vi "SVA 4MV6 P001 CCE.vi"() -> ()   [LabVIEW 2020]
doc: "Ceballos Conde Emanuel 4MV6 Sistemas de visión artificial 2022/1\nEste vi permite obtener el gradiente en x , gradiente en Y o gradiente general en susecion de una serie de imagenes ubicadas en una carpeta , si se utiliza como subvi la salida obtenida sera el gradiente da la ultima imagen de la carpeta."
uses:
  <vilib>/userDefined/High Color/IMAQdx.ctl
  <vilib>/vision/driver/IMAQdx.llb/IMAQdx Buffer Number Mode.ctl
  <vilib>/vision/driver/NI_Vision_Acquisition_Software.lvlib
panel:
  out "Cal Dis":bool
  out "CII":bool
  out "CID":bool
  in  "recalcular distancia":bool
  in  "recapturar imagen izquierda":bool
  in  "recapturar Imagen derecha":bool
  in  "capturar":bool
  out "Imagen izquierda":T1(plugin-control)
  out "video":T1(plugin-control)
  in  "stop":bool
  in  "Session In":T2
  out "Bcx":u32
  out "Bcy":u32
  out "Gcx":u32
  out "Gcy":u32
  out "Rcy":u32
  out "Rcx":u32
  out "Imagen derecha":T1(plugin-control)
  # "Ceballos Conde Emanuel\n4MV6\nSistemas de visión artificial\n2022/1"
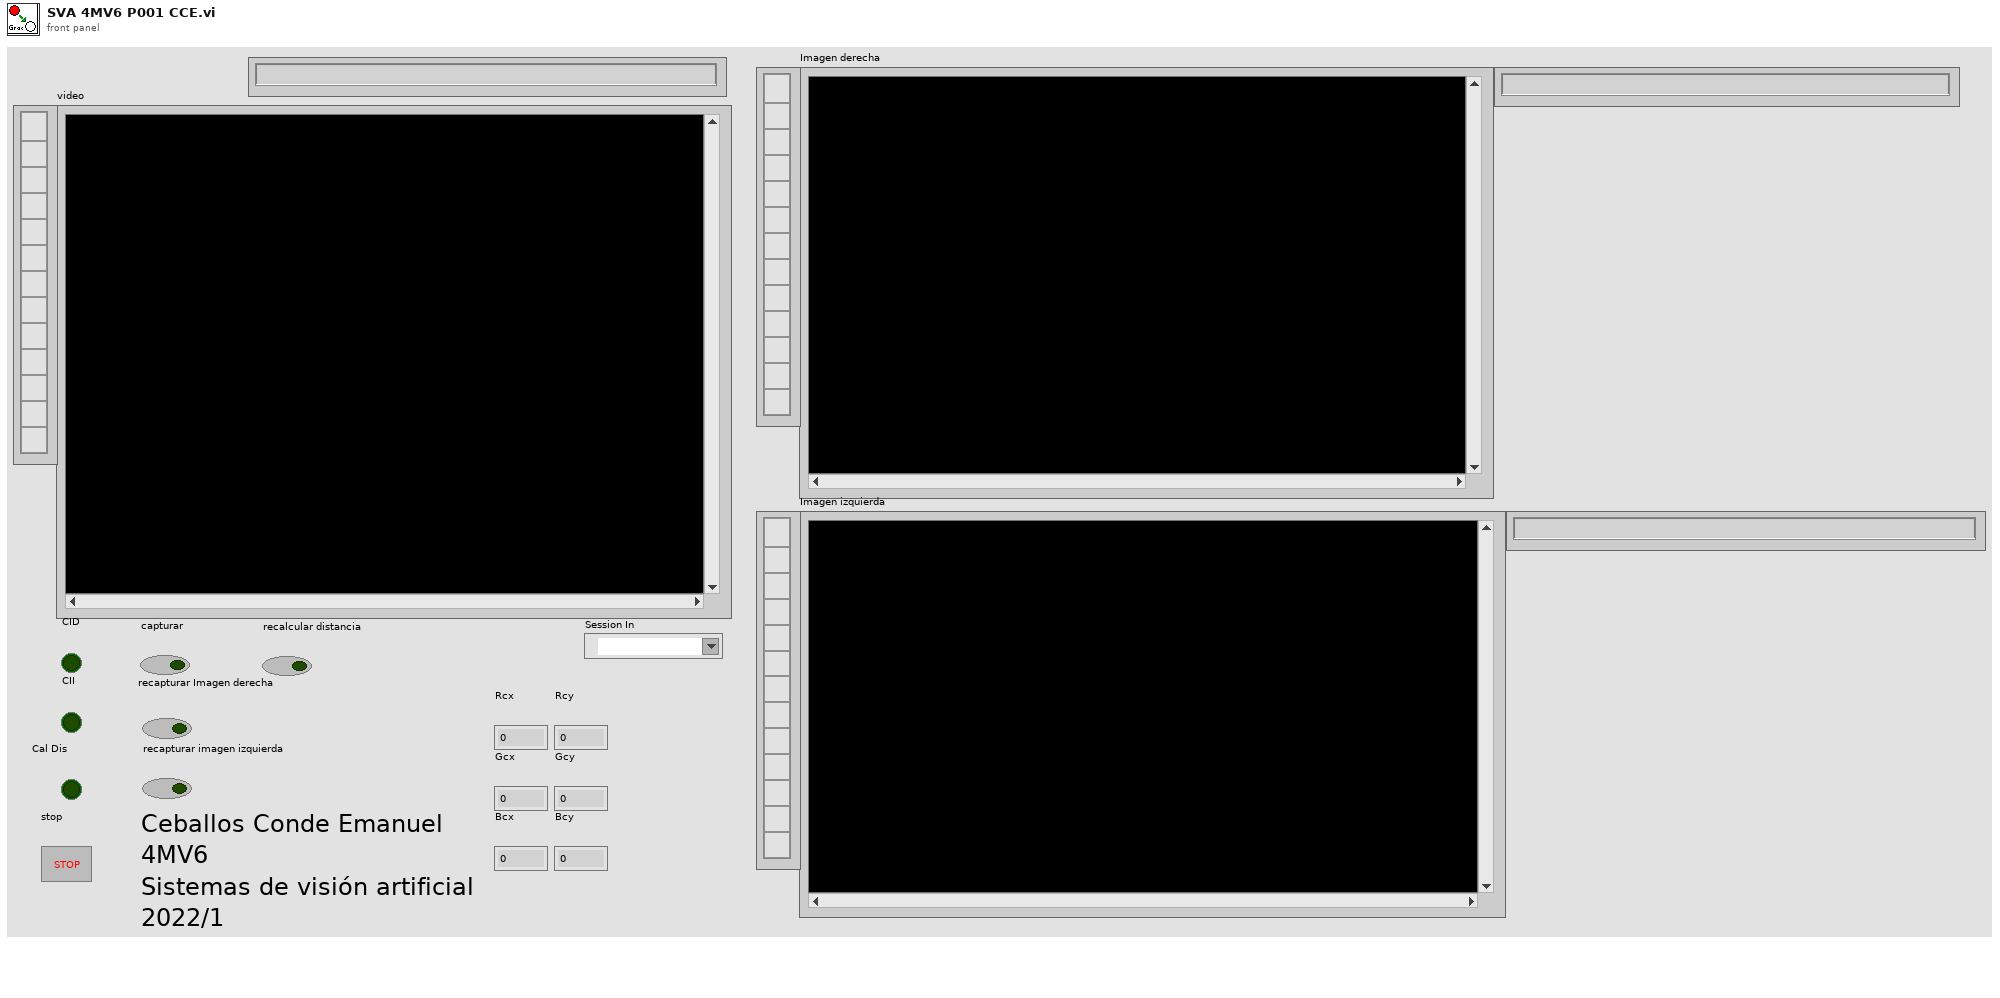
[diagram p1: front panel]
types:
  T1 = typedef "IMAQ Image.ctl" = refnum<image>
  T2 = typedef "IMAQdx.ctl" = refnum<k21>
  T3 = typedef "Image Type" = u32
  T4 = enum16{"captura imagen derecha", "captura imagen izquierda", "calculo de distancia"}
  T5 = typedef "NI_Vision_Acquisition_Software.lvlib/IMAQdx Buffer Number Mode.ctl" = enum32{"Next", "Last", "Buffer Number", "Every", "Last New"}
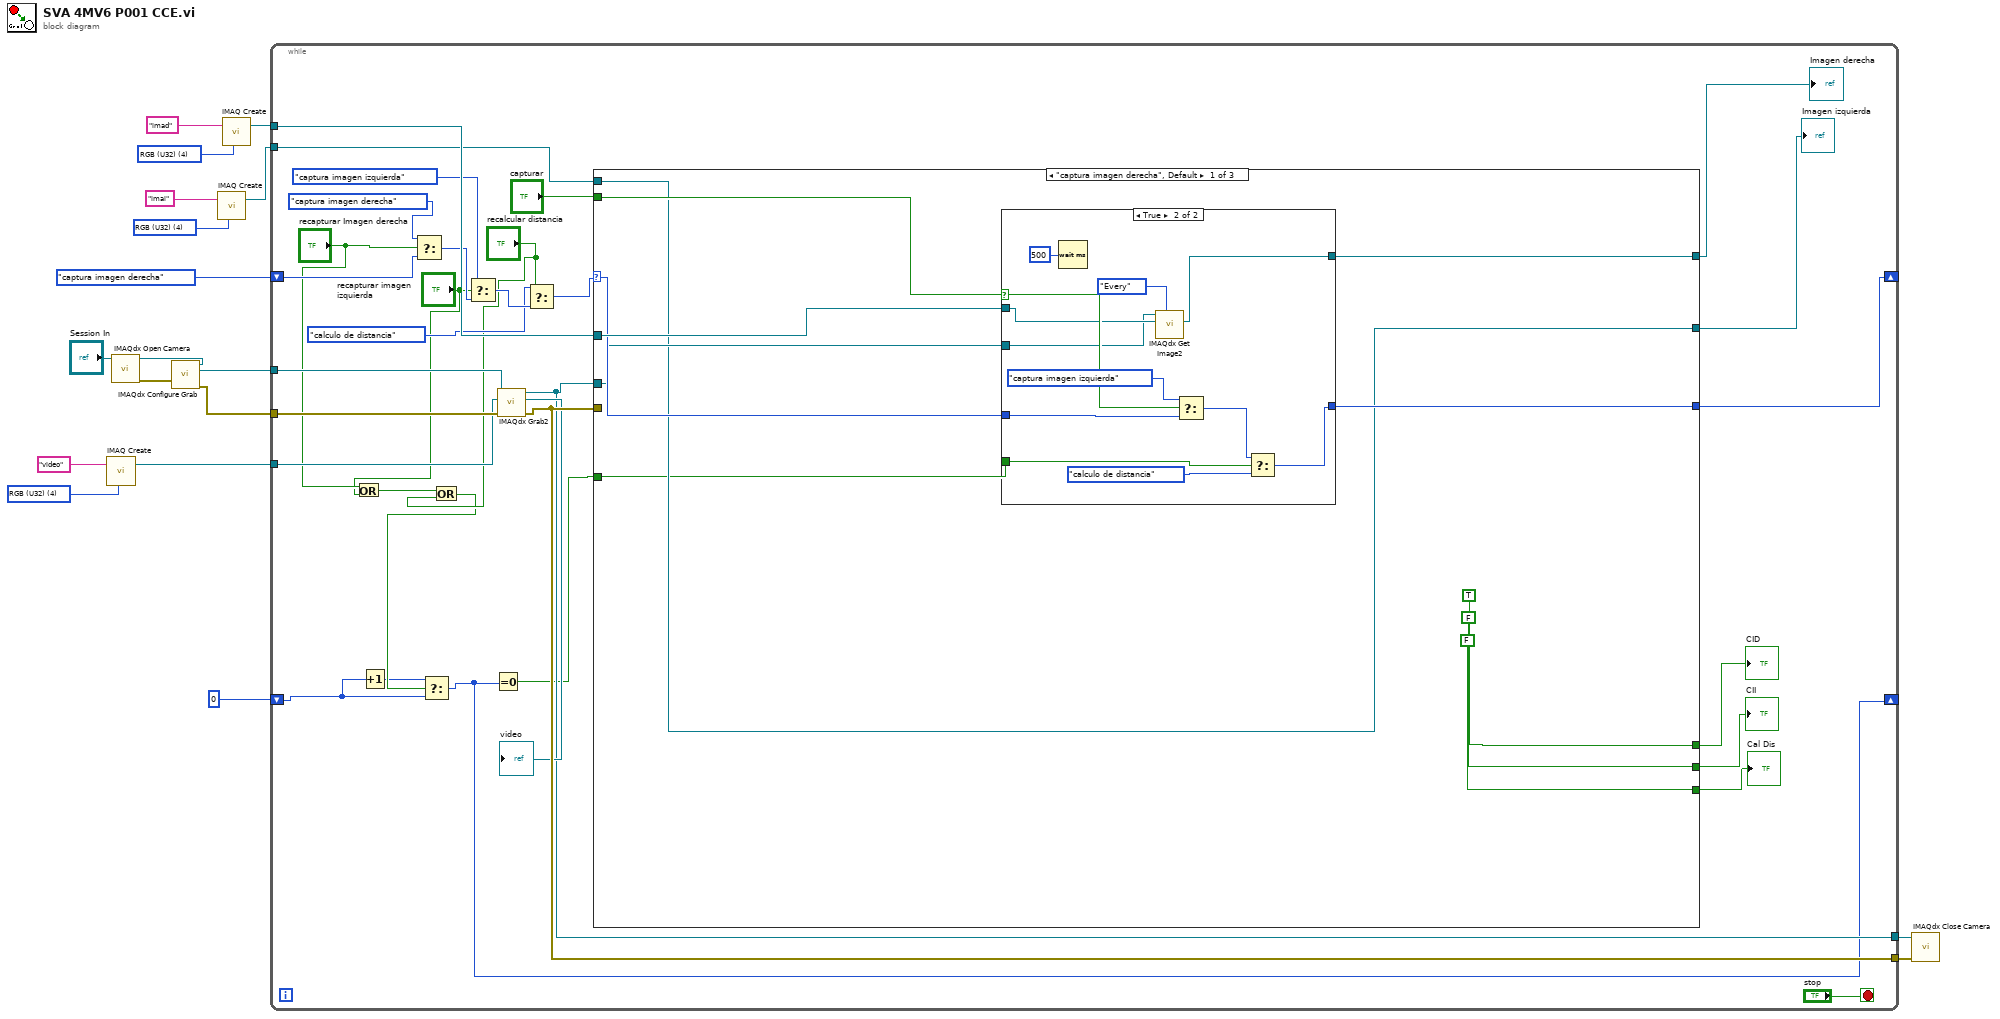
[diagram p0: block diagram]
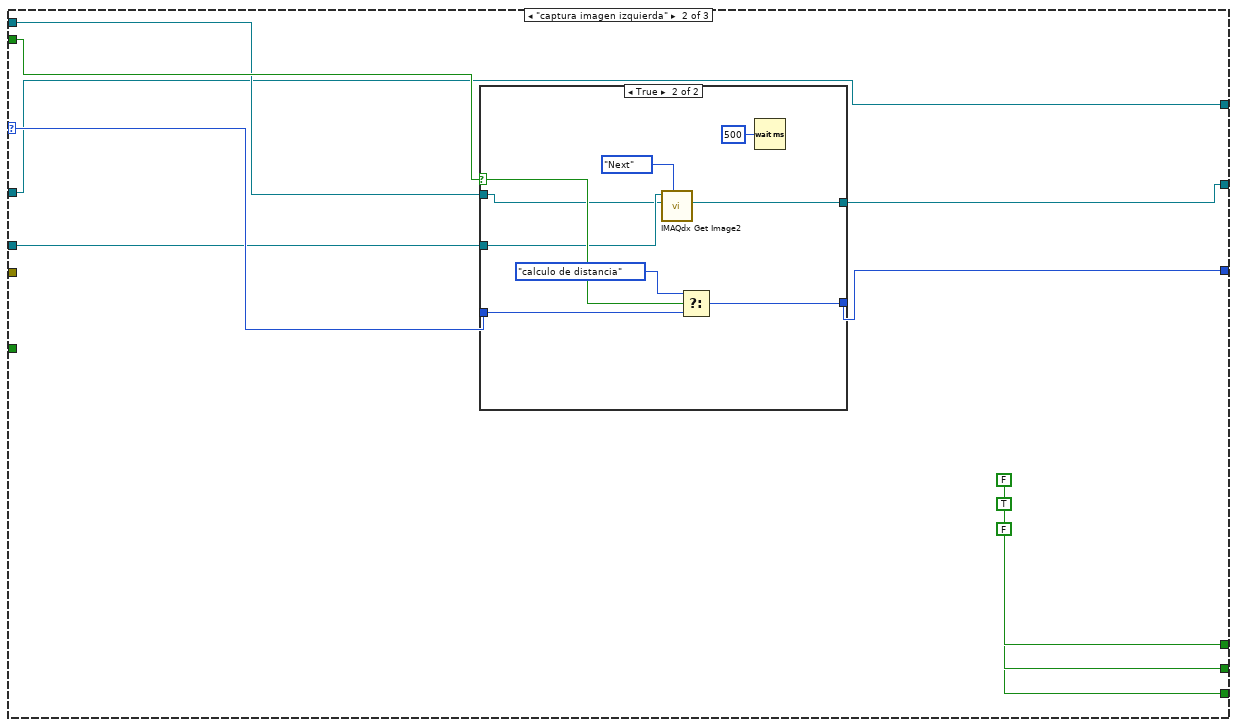
[diagram p3: hidden frame]
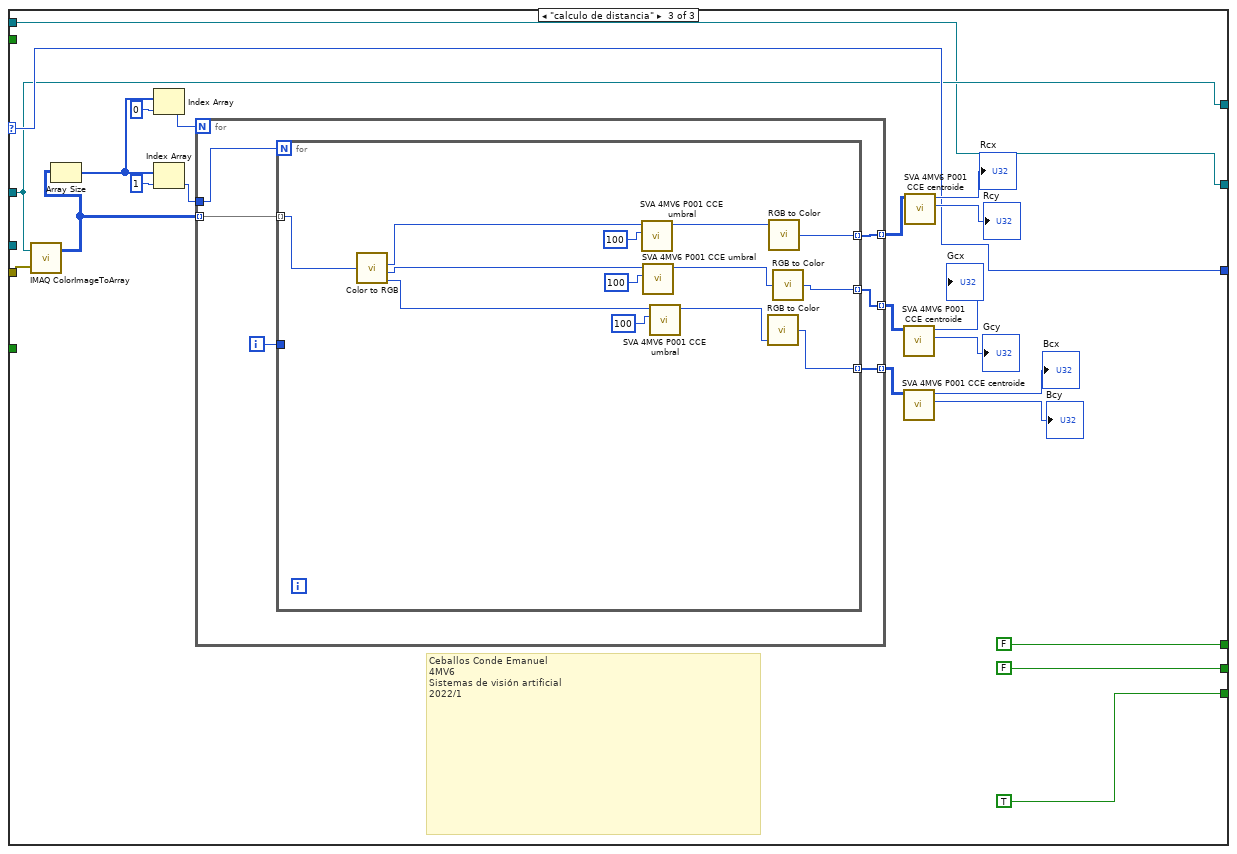
[diagram p5: hidden frame]
diagram:
  w3 = T3 4 items=["Grayscale (U8)", "Grayscale (I16)", "Grayscale (SGL)", "Complex (CSG)", "RGB (U32)", "HSL (U32)", "RGB (U64)", "Grayscale (U16)"] ("Image Type")
  w11 = T3 4 items=["Grayscale (U8)", "Grayscale (I16)", "Grayscale (SGL)", "Complex (CSG)", "RGB (U32)", "HSL (U32)", "RGB (U64)", "Grayscale (U16)"] ("Image Type")
  w16 = T3 4 items=["Grayscale (U8)", "Grayscale (I16)", "Grayscale (SGL)", "Complex (CSG)", "RGB (U32)", "HSL (U32)", "RGB (U64)", "Grayscale (U16)"] ("Image Type")
  n1 = call "IMAQ Create"("Image Name"="video", "Image Type"=w11) -> ("New Image"=w8:T1)  [unwired: 3 in, 1 out]
  n2 = call <vilib>:"IMAQdx Open Camera.vi"("Session In"="Session In") -> ("error out"=w14:errorcluster, "Session Out"=w15:T2)  [unwired: 9 in]
  n3 = call <vilib>:"IMAQdx Configure Grab.vi"("error in"=w14, "Session In"=w15) -> ("error out"=w9:errorcluster, "Session Out"=w10:T2)  [unwired: 8 in]
  n4 = call "IMAQ Create"("Image Name"="imai", "Image Type"=w3) -> ("New Image"=w2:T1)  [unwired: 3 in, 1 out]
  n5 = call "IMAQ Create"("Image Name"="imad", "Image Type"=w16) -> ("New Image"=w18:T1)  [unwired: 3 in, 1 out]
  n6 = while {
    tunnel: w10 -> [w50]
    tunnel: w9 -> [w49]
    tunnel: w8 -> [w48]
    tunnel: [w42] -> w7
    tunnel: [w46] -> w6
    shift-right: [w41] -> _
    shift-left: T4."captura imagen derecha" ("Método") -> [w39]
    tunnel: w18 -> [w43]
    tunnel: w2 -> [w33]
    shift-right: [w19] -> _
    shift-left: 0 -> [w22]
    stop <- "stop" stop-if-true
    n7 = Or(x="recapturar Imagen derecha", y="recapturar imagen izquierda") -> (x .or. y?=w27:bool)
    n8 = Increment(x=w22) -> (x+1=w21:i32)
    n9 = Select(t=T4."captura imagen derecha" ("Método"), s="recapturar Imagen derecha", f=w39) -> (s? t:f=w40:T4)
    n10 = Or(x=w27, y="recalcular distancia") -> (x .or. y?=w23:bool)
    n11 = Select(t=w21, s=w23, f=w22) -> (s? t:f=w19:i32)
    n12 = Select(t=T4."captura imagen izquierda" ("Método"), s="recapturar imagen izquierda", f=w40) -> (s? t:f=w36:T4)
    n13 = Equal To 0?(x=w19) -> (x = 0?=w20:bool)
    n14 = call <vilib>:"IMAQdx Grab2.vi"("error in"=w49, "Image In"=w48, "Session In"=w50) -> ("error out"=w46:errorcluster, "Image Out"=→"video":T1, "Session Out"=w42:T2)  [unwired: 5 in, 1 out]
    n15 = Select(t=T4."calculo de distancia" ("Método"), s="recalcular distancia", f=w36) -> (s? t:f=w35:T4)
    n16 = case shown="\"captura imagen derecha\", Default" w35 {
      selector: w35 -> [w58 w84 w102]
      tunnel: w46 -> [_ _ w115]
      tunnel: "capturar" -> [w61 w85 _]
      tunnel: w43 -> [w60 w79 w101]
      tunnel: w42 -> [w57 w81 _]
      tunnel: [w59 w83 w102] -> w41
      tunnel: w33 -> [w55 w82 w100]
      tunnel: [w56 w79 w101] -> w32
      tunnel: [w55 w80 w100] -> w31
      tunnel: [TRUE ("CID") FALSE ("CID") FALSE ("CID")] -> w30
      tunnel: [FALSE ("CID") TRUE ("CID") FALSE ("CID")] -> w29
      tunnel: [FALSE ("CID") FALSE ("CID") TRUE ("CID")] -> w28
      tunnel: w20 -> [w51 _ _]
      frame "captura imagen derecha", Default {
        n17 = case shown="True" w61 {
          selector: w61 -> [_ w75]
          tunnel: w60 -> [w62 w72]
          tunnel: [w63 w67] -> w59
          tunnel: w58 -> [w63 w73]
          tunnel: w57 -> [_ w71]
          tunnel: [w62 w69] -> w56
          tunnel: w51 -> [_ w64]
          frame False {
          }
          frame True {
            n18 = Wait (ms)(milliseconds to wait=u32 500) -> ()  [unwired: 1 out]
            n19 = call <vilib>:"IMAQdx Get Image2.vi"("Buffer Number Mode (Next)"=IMAQdx_Buffer_Number_Mode."Every", "Image In"=w72, "Session In"=w71) -> ("Image Out"=w69:T1)  [unwired: 5 in, 3 out]
            n20 = Select(t=T4."captura imagen izquierda" ("Método"), s=w75, f=w73) -> (s? t:f=w65:T4)
            n21 = Select(t=w65, s=w64, f=T4."calculo de distancia" ("Método")) -> (s? t:f=w67:T4)
          }
        }
      }
      frame "captura imagen izquierda" {
        n22 = case shown="True" w85 {
          selector: w85 -> [_ w95]
          tunnel: w82 -> [w86 w91]
          tunnel: [w87 w96] -> w83
          tunnel: w84 -> [w87 w93]
          tunnel: w81 -> [_ w92]
          tunnel: [w86 w89] -> w80
          frame False {
          }
          frame True {
            n23 = call <vilib>:"IMAQdx Get Image2.vi"("Buffer Number Mode (Next)"=IMAQdx_Buffer_Number_Mode."Next", "Image In"=w91, "Session In"=w92) -> ("Image Out"=w89:T1)  [unwired: 5 in, 3 out]
            n24 = Select(t=T4."calculo de distancia" ("Método"), s=w95, f=w93) -> (s? t:f=w96:T4)
            n25 = Wait (ms)(milliseconds to wait=u32 500) -> ()  [unwired: 1 out]
          }
        }
      }
      frame "calculo de distancia" {
        # "Ceballos Conde Emanuel\n4MV6\nSistemas de visión artificial\n2022/1"
        n26 = call "IMAQ ColorImageToArray"("Image"=w101, "error in (no error)"=w115) -> ("Image Pixels (U32)"=w116:u32[][])  [unwired: 2 in, 2 out]
        n27 = Array Size(array=w116) -> (size(s)=w118:i32[])
        n28 = Index Array(array=w118, index=0) -> (element=w114:i32)
        n29 = Index Array(array=w118, index=1) -> (element=w112:i32)
        n30 = for {
          N: w114 -> [_]
          tunnel: w116 -> [w124] mode=indexing
          tunnel: [w122] -> w117 mode=indexing
          tunnel: w112 -> [w121]
          tunnel: [w120] -> w103 mode=indexing
          tunnel: [w119] -> w104 mode=indexing
          i -> [w123]
          n31 = for {
            N: w121 -> [_]
            tunnel: w124 -> [w137] mode=indexing
            tunnel: w123 -> [_]
            tunnel: [w129] -> w122 mode=indexing
            tunnel: [w126] -> w120 mode=indexing
            tunnel: [w125] -> w119 mode=indexing
            n32 = call <vilib>:"Color to RGB.vi"("Color"=w137) -> ("R"=w131:u8, "G"=w132:u8, "B"=w135:u8)  [unwired: 1 out]
            n33 = call "SVA 4MV6 P001 CCE umbral.vi"("gris"=w131, "umbral"=u8 100) -> ("umbralizado"=w130:u8)  [unwired: 8 in]
            n34 = call "SVA 4MV6 P001 CCE umbral.vi"("gris"=w132, "umbral"=u8 100) -> ("umbralizado"=w128:u8)  [unwired: 8 in]
            n35 = call "SVA 4MV6 P001 CCE umbral.vi"("gris"=w135, "umbral"=u8 100) -> ("umbralizado"=w127:u8)  [unwired: 8 in]
            n36 = call <vilib>:"RGB to Color.vi"("B"=w127) -> ("Color"=w125:u32)  [unwired: 2 in]
            n37 = call <vilib>:"RGB to Color.vi"("R"=w130) -> ("Color"=w129:u32)  [unwired: 2 in]
            n38 = call <vilib>:"RGB to Color.vi"("G"=w128) -> ("Color"=w126:u32)  [unwired: 2 in]
          }
        }
        n39 = call "SVA 4MV6 P001 CCE centroide .vi"("Array"=w103) -> ("cy"=→"Gcy":u32, "cx"=→"Gcx":u32)  [unwired: 9 in]
        n40 = call "SVA 4MV6 P001 CCE centroide .vi"("Array"=w104) -> ("cy"=→"Bcy":u32, "cx"=→"Bcx":u32)  [unwired: 9 in]
        n41 = call "SVA 4MV6 P001 CCE centroide .vi"("Array"=w117) -> ("cy"=→"Rcy":u32, "cx"=→"Rcx":u32)  [unwired: 9 in]
      }
    }
    "Imagen derecha" <- w32
    "Imagen izquierda" <- w31
    "CID" <- w30
    "Cal Dis" <- w28
    "CII" <- w29
  }
  n42 = call <vilib>:"IMAQdx Close Camera.vi"("error in"=w6, "Session In"=w7) -> ()  [unwired: 9 in, 1 out]
